vi "dfd_SRate G Check File Existence.vi"(5 "code type":u16(ring) items=["Integer LabVIEW", "LabVIEW FPGA"], 6 "confirm?":bool=TRUE, 7 "# channels":i32=1, 8 "error in (no error)":errorcluster, 9 "filter name":string, 10 "dest path":path, 11 "filter in":T1={"mSRate_Fs"=1.0, "mSRate_Version"="1.0", "mSRate_Comments"="", "mSRate_OrgCoef"={"type"=enum."Undefined", "gain"=1.0, "coef a (k)"=[], "coef b (v)"=[]}, "mSRate_CurCoef"={"type"=enum."Undefined", "gain"=1.0, "coef a (k)"=[], "coef b (v)"=[]}, "mSRate_Quantized?"=FALSE, "mSRate_QCoef"={"type"=enum."Undefined", "gain"=1.0, "coef a (k)"=[], "coef b (v)"=[]}, "mSRate_QSettings"=[], "mSRate_Order"=0, "mSRate_Scaling"={"mSRate_ScaleByPowerOf2?"=FALSE, "mSRate_ScaleType"=enum."No Norm"}} {"mSRate_QSettings"."source" items=["Coef a/k"=0, "Coef b/v"=7, "Input"=1, "Output"=2, "Multiplicand"=3, "Product"=4, "Sum"=5, "Delay"=6, "Gain"=8]}) -> (0 "error out":errorcluster, 1 "filter name out":string)   [LabVIEW 2017, in "NI_DigFilterLicensed.lvlib"]
uses:
  <vilib>/addons/Digital Filter Design/NI_DigFilterLicensed.lvlib
  <vilib>/addons/Digital Filter Design/_Objects.llb/DFD Filter Obj.ctl
  <vilib>/addons/Digital Filter Design/_Objects.llb/DFD Filter Coef.ctl
  <vilib>/addons/Digital Filter Design/_Objects.llb/DFD Filter Structure Type Selector.ctl
  <vilib>/addons/Digital Filter Design/_Objects.llb/dfd_Internal Quantization Settings.ctl
  <vilib>/addons/Digital Filter Design/_Objects.llb/dfd_Internal Quantization Srcs.ctl
  <vilib>/addons/Digital Filter Design/_Objects.llb/DFD Coef Norm Type.ctl
  <vilib>/addons/Digital Filter Design/_Misc.llb/dfd_Error Handlers (Single).vi
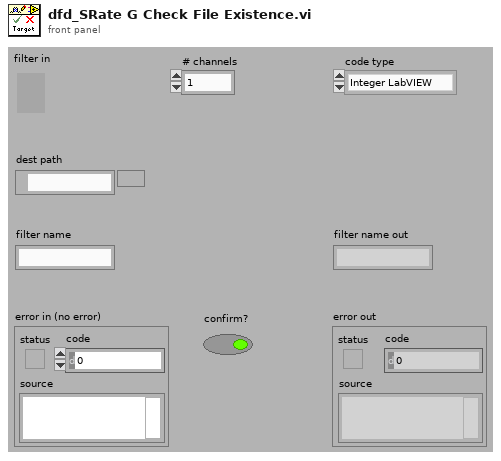
[diagram p1: front panel]
types:
  T1 = typedef "NI_DigFilterLicensed.lvlib/DFD Filter Obj.ctl" = cluster{"mSRate_Fs":dbl, "mSRate_Version":string, "mSRate_Comments":string, "mSRate_OrgCoef":T2, "mSRate_CurCoef":T2, "mSRate_Quantized?":bool, "mSRate_QCoef":T2, "mSRate_QSettings":T4[], "mSRate_Order":i32, "mSRate_Scaling":cluster{"mSRate_ScaleByPowerOf2?":bool, "mSRate_ScaleType":T6}}
  T2 = typedef "NI_DigFilterLicensed.lvlib/DFD Filter Coef.ctl" = cluster{"type":T3, "gain":dbl, "coef a (k)":dbl[], "coef b (v)":dbl[]}
  T3 = typedef "NI_DigFilterLicensed.lvlib/DFD Filter Structure Type Selector.ctl" = enum16{"Undefined", "FIR Direct Form", "FIR Direct Form Transposed", "FIR Symmetric", "FIR Antisymmetric", "IIR Direct Form I", "IIR Direct Form I Transposed", "IIR Direct Form II", "IIR Direct Form II Transposed", "IIR Cascaded Second Order Sections Form I", "IIR Cascaded Second Order Sections Form I Transposed", "IIR Cascaded Second Order Sections Form II", "IIR Cascaded Second Order Sections Form II Transposed", "Lattice Allpass (basic sections)", "Lattice Allpass (one multiplier sections)", "Lattice Allpass (normalized sections)", "Lattice AR (basic sections)", "Lattice AR (one multiplier sections)", "Lattice AR (normalized sections)", "Lattice MA (minimum phase)", "Lattice MA (maximum phase)", "Lattice ARMA (basic sections)", "Lattice ARMA (one multiplier sections)", "Lattice ARMA (normalized sections)"}
  T4 = typedef "NI_DigFilterLicensed.lvlib/dfd_Internal Quantization Settings.ctl" = cluster{"source":T5, "wl":i16, "iwl":i16, "overflow mode":enum16{"Saturation", "Wrap"}, "rounding mode":enum16{"Nearest", "Truncation"}, "signed?":bool}
  T5 = typedef "NI_DigFilterLicensed.lvlib/dfd_Internal Quantization Srcs.ctl" = u16
  T6 = typedef "NI_DigFilterLicensed.lvlib/DFD Coef Norm Type.ctl" = enum16{"No Norm", "Time Domain 1-Norm", "Time Domain 2-Norm", "Time Domain Inf-Norm"}
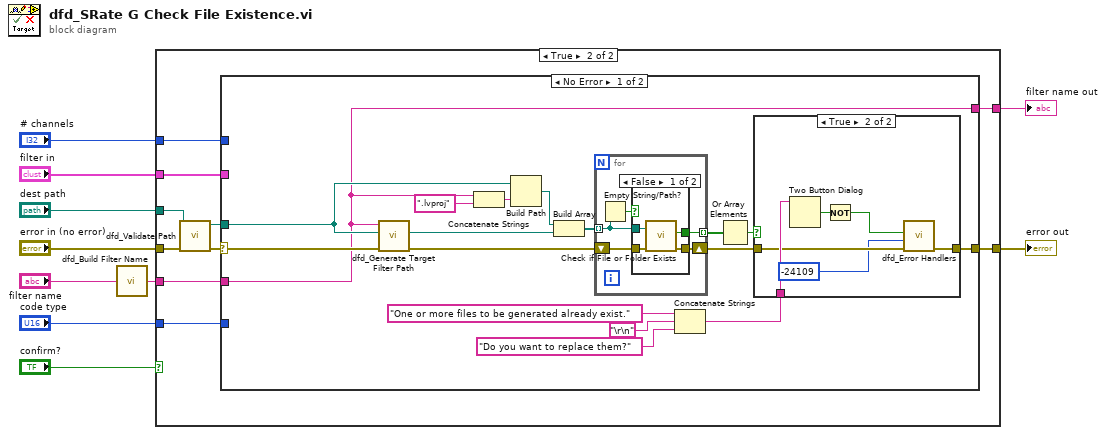
[diagram p0: block diagram]
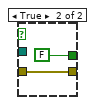
[diagram p4: hidden frame]
diagram:
  n1 = call <vilib>:"dfd_Build Filter Name.vi"("filter name in"="filter name") -> ("filter name out"=w1:string)
  n2 = case shown="True" "confirm?" {
    tunnel: "error in (no error)" -> [w12 w22]
    tunnel: "dest path" -> [_ w21]
    tunnel: w1 -> [w11 w20]
    tunnel: [w11 w18] -> w8
    tunnel: [w12 w16] -> w7
    tunnel: "filter in" -> [_ w15]
    tunnel: "# channels" -> [_ w14]
    tunnel: "code type" -> [_ w13]
    frame False {
    }
    frame True {
      n3 = call <vilib>:"dfd_Validate Path.vi"("error in (no error)"=w22, "path in"=w21) -> ("error out"=w17:errorcluster, "path out"=w19:path)  [unwired: 8 out]
      n4 = case shown="No Error" w17 {
        selector: w17 -> [w39 w59]
        tunnel: w20 -> [w23 w58]
        tunnel: w19 -> [w36 _]
        tunnel: [w23 w58] -> w18
        tunnel: [w27 w59] -> w16
        tunnel: w15 -> [_ _]
        tunnel: w14 -> [_ _]
        tunnel: w13 -> [_ _]
        frame No Error {
          n5 = call <vilib>:"dfd_Generate Target Filter Path.vi"("error in (no error)"=w39, "destination path"=w36, "filter name"=w23) -> ("error out"=w28:errorcluster, "target VI path"=w34:path)  [unwired: 3 in, 4 out]
          n6 = Concatenate Strings(w23, ".lvproj" ("string")) -> (w37:string)
          n7 = Build Path(base path=w36, name or relative path=w37) -> (appended path=w35:path)
          n8 = Build Array(w35, w34) -> (w26:path[])
          n9 = for {
            tunnel: w26 -> [w48] mode=indexing
            shift-right: [w50] -> w31
            shift-left: w28 -> [w51]
            tunnel: [w49] -> w33 mode=indexing
            n10 = Empty String/Path?(string/path=w48) -> (empty?=w47:bool)
            n11 = case shown="False" w47 {
              tunnel: w51 -> [w55 w56]
              tunnel: w48 -> [w54 _]
              tunnel: [w53 w56] -> w50
              tunnel: [w52 FALSE ("file or folder exists?")] -> w49
              frame False {
                n12 = call <vilib>:"Check if File or Folder Exists.vi"("error in (no error)"=w55, "path"=w54) -> ("error out"=w53:errorcluster, "file or folder exists?"=w52:bool)  [unwired: 8 out]
              }
              frame True {
              }
            }
          }
          n13 = Concatenate Strings("One or more files to be generated already exist.", "\r\n", "Do you want to replace them?") -> (w29:string)
          n14 = Or Array Elements(Boolean array=w33) -> (logical OR=w32:bool)
          n15 = case shown="True" w32 {
            tunnel: w31 -> [w40 w45]
            tunnel: w29 -> [_ w46]
            tunnel: [w40 w44] -> w27
            frame False {
            }
            frame True {
              n16 = Two Button Dialog(message=w46) -> (T button?=w43:bool)  [unwired: 2 out]
              n17 = Not(x=w43) -> (.not. x?=w42:bool)
              n18 = call-poly <vilib>:"dfd_Error Handlers.vi"("error in (no error)"=w45, "error code"=-24109 ("ERR_CODEGEN_CANCELLED"), "condition failed?"=w42) -> ("error out"=w44:errorcluster)  [unwired: 8 out]
            }
          }
        }
        frame Error {
        }
      }
    }
  }
  "error out" <- w7
  "filter name out" <- w8
